vi "Invoice History.vi"(11 "reference in":T1) -> (3 "reference out":T1)   [LabVIEW 2017]
uses:
  <vilib>/addons/database/Connection.llb/Conn ObjectReference.ctl
  Control/State machine.ctl
  <vilib>/Utility/miscctls.llb/LVPointTypeDef.ctl
  8dd361f1-169d-4dbd-a915-f8e7e06827b6.vi
  <vilib>/Array/Sort 2D Array - Pop Stack.vi
  <vilib>/Array/Sort 2D Array - Push Stack.vi
  <vilib>/addons/database/Connection.llb/Conn Execute.vi
  <vilib>/addons/database/Recordset.llb/Rec Fetch Recordset Data (R).vi
  <vilib>/addons/database/Recordset.llb/Rec Destroy - Connection.vi
  <vilib>/addons/database/_DB Variant To Data/Database Variant To Data.xnode
  <vilib>/addons/database/NI_Database_API.lvlib
panel:
  in  "Search":string(combo)
  in  "Invoice CODE":string(combo)
  out "Invoice Date":timestamp format="%<%d/%m/%Y>T"
  out "Table":string[][](table)
  # "INVOICE HISTORY"
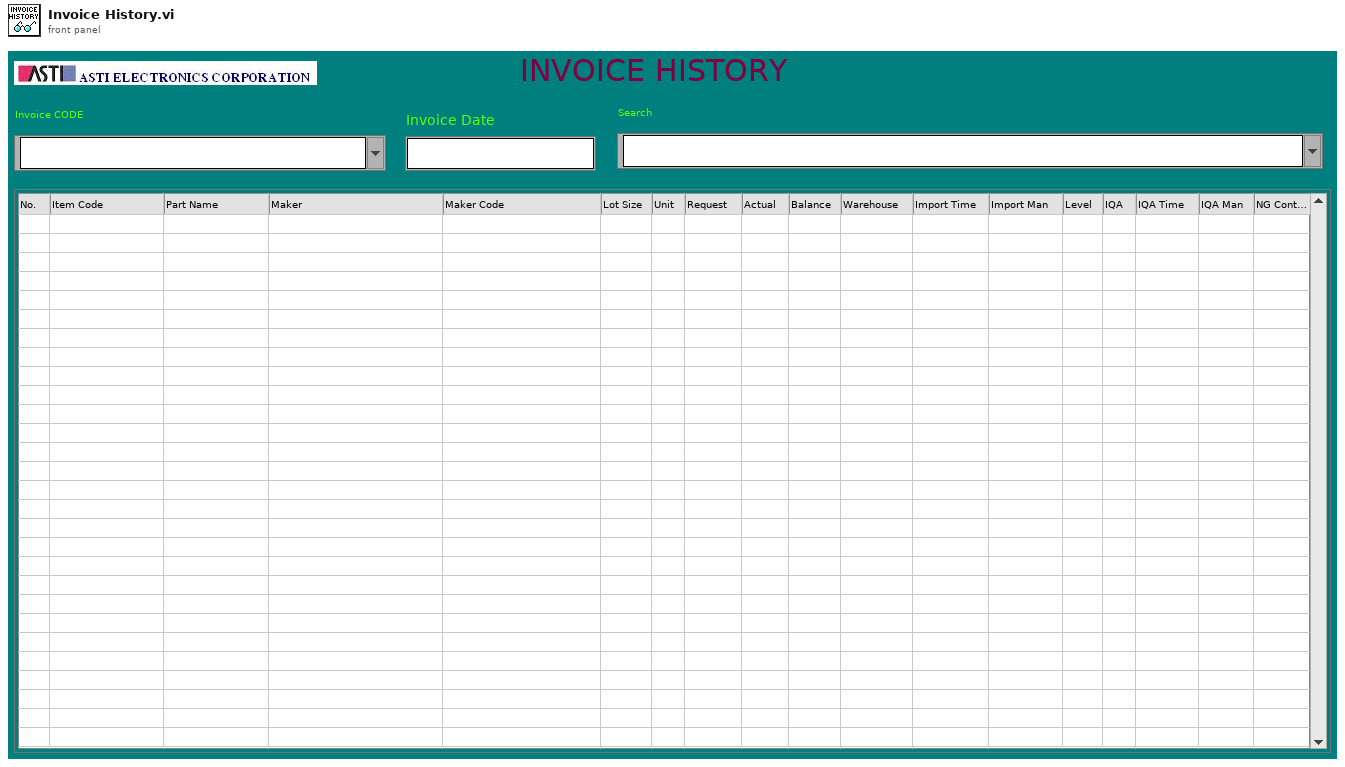
[diagram p1: front panel]
types:
  T1 = typedef "NI_Database_API.lvlib/Conn ObjectReference.ctl" = refnum<k1>
  T2 = typedef "LVPointTypeDef.ctl" = cluster{"Horizontal":i16, "Vertical":i16}
  T3 = typedef "State machine.ctl" = enum16{"Licence check", "Initial", "Log in", "Creat Config file", "Network setting", "Creat database 1", "Creat database 2", "Creat database 3", "Transfer", "Begin", "Exit"}
  T4 = typedef "NI_Database_API.lvlib/Rec ObjectReference.ctl" = refnum<k1>
  T5 = cluster{"[0]":string, "[1]":string, "[2]":string, "[3]":string, "[4]":string, "[5]":string, "[6]":string, "[7]":string, "[8]":string, "[9]":string, "[10]":string, "[11]":string, "[12]":string, "[13]":string, "[14]":string, "[15]":string}
  T6 = cluster{"[0]":string, "[1]":string, "[2]":string, "[3]":string, "[4]":string, "[5]":string, "[6]":string, "[7]":string, "[8]":string, "[9]":string, "[10]":string, "[11]":string, "[12]":string, "[13]":string, "[14]":string, "[15]":string}[]
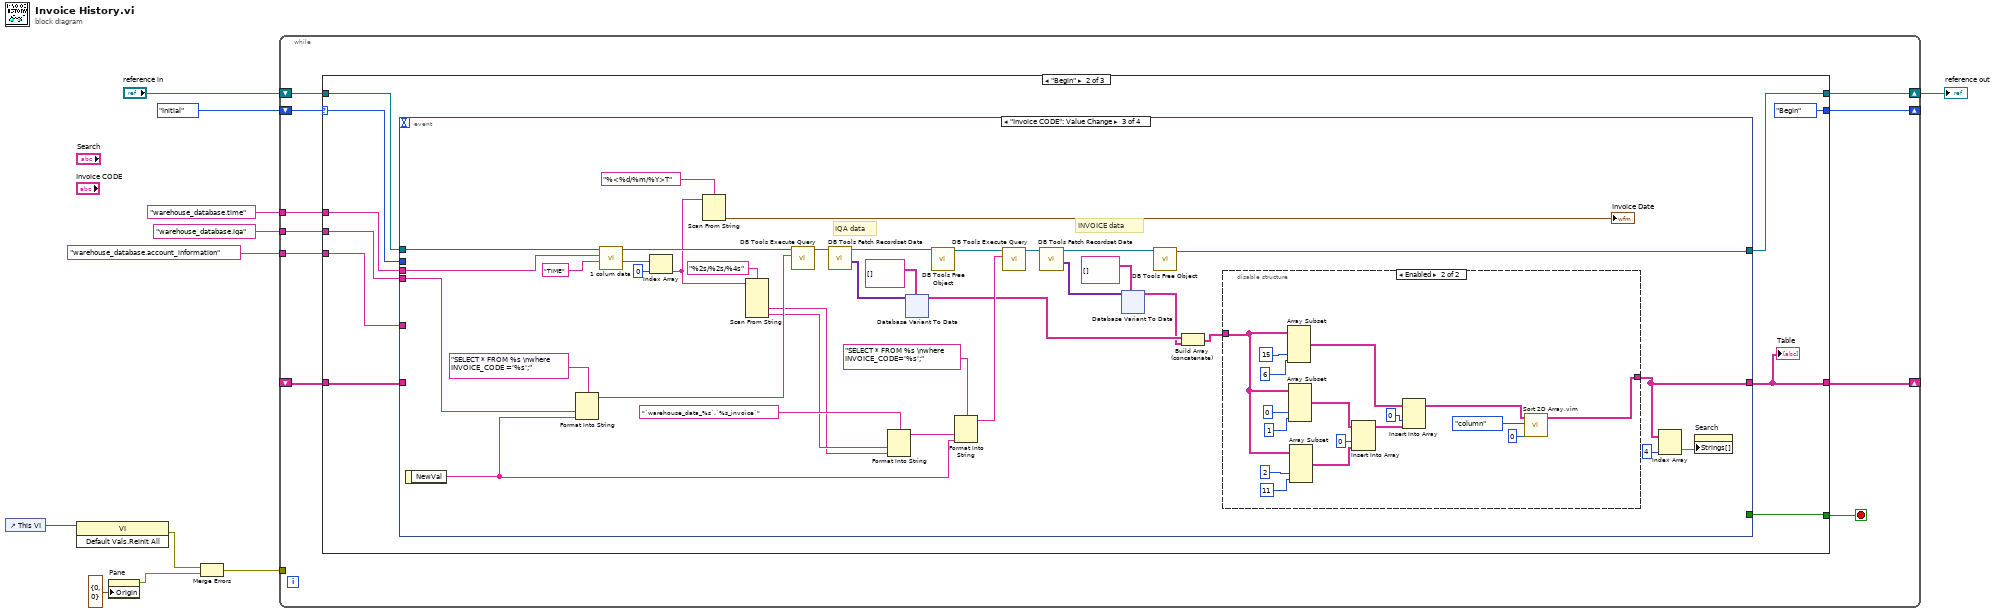
[diagram p0: block diagram]
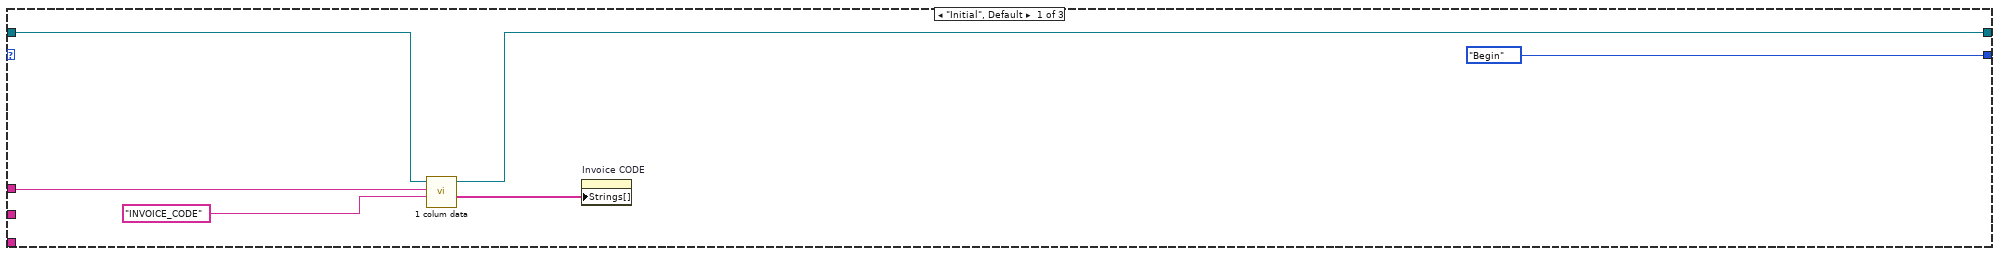
[diagram p2: hidden frame]
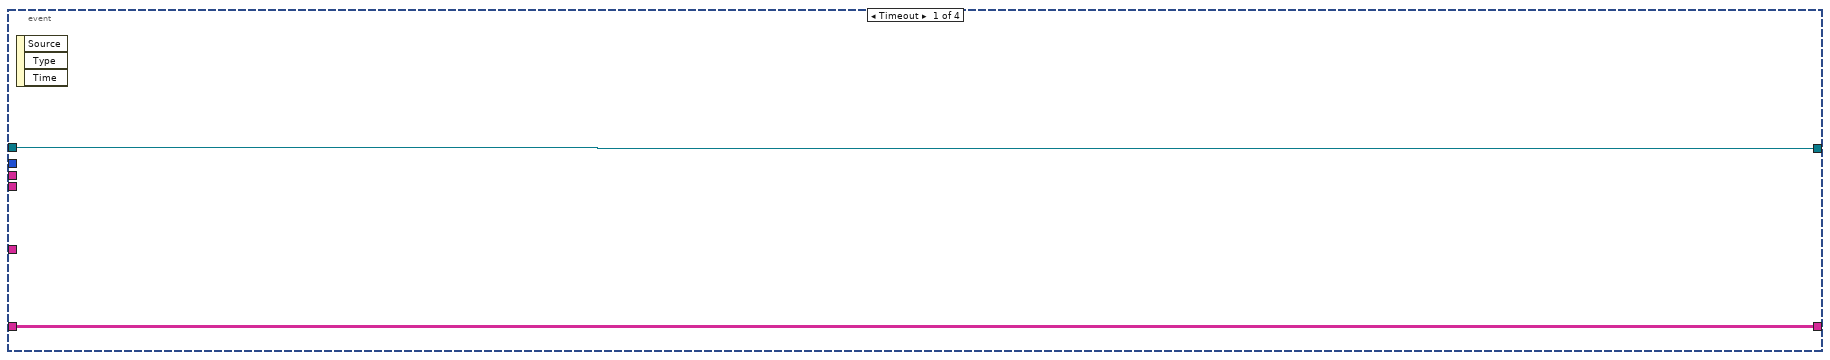
[diagram p3: hidden frame]
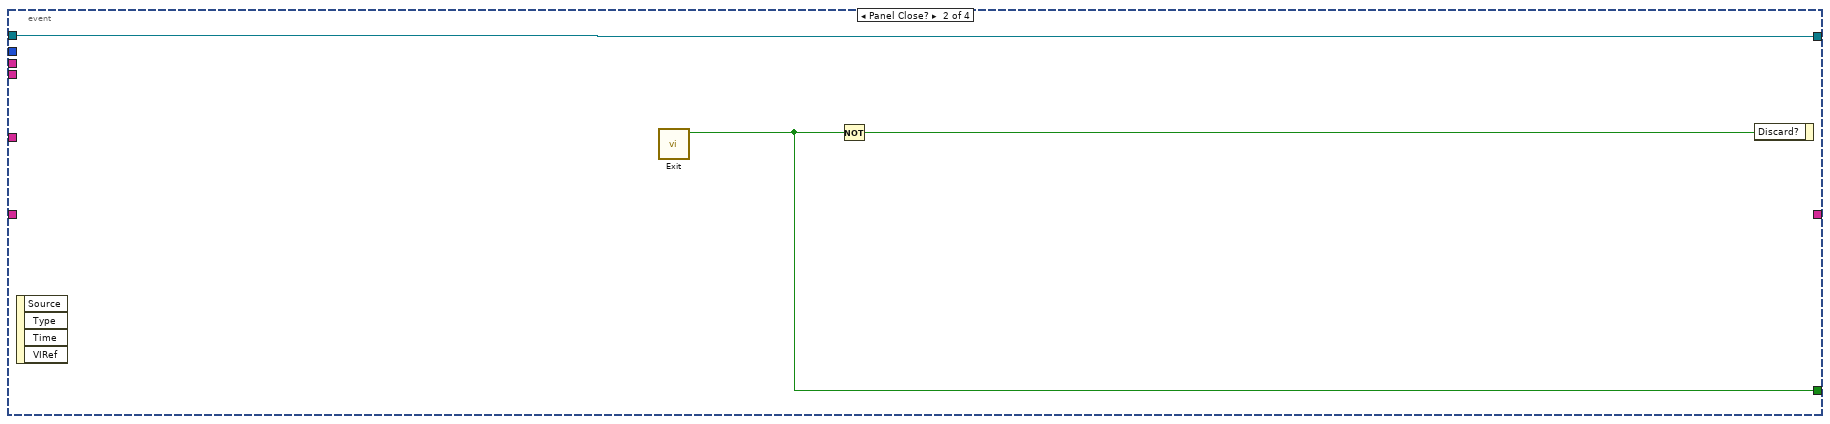
[diagram p4: hidden frame]
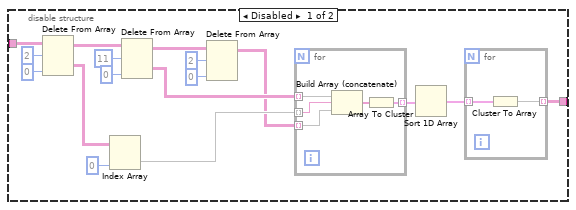
[diagram p5: hidden frame]
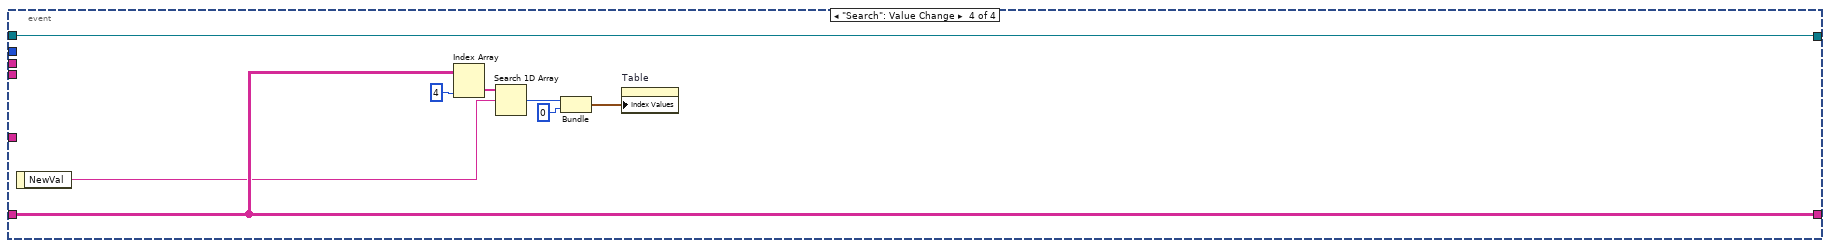
[diagram p6: hidden frame]
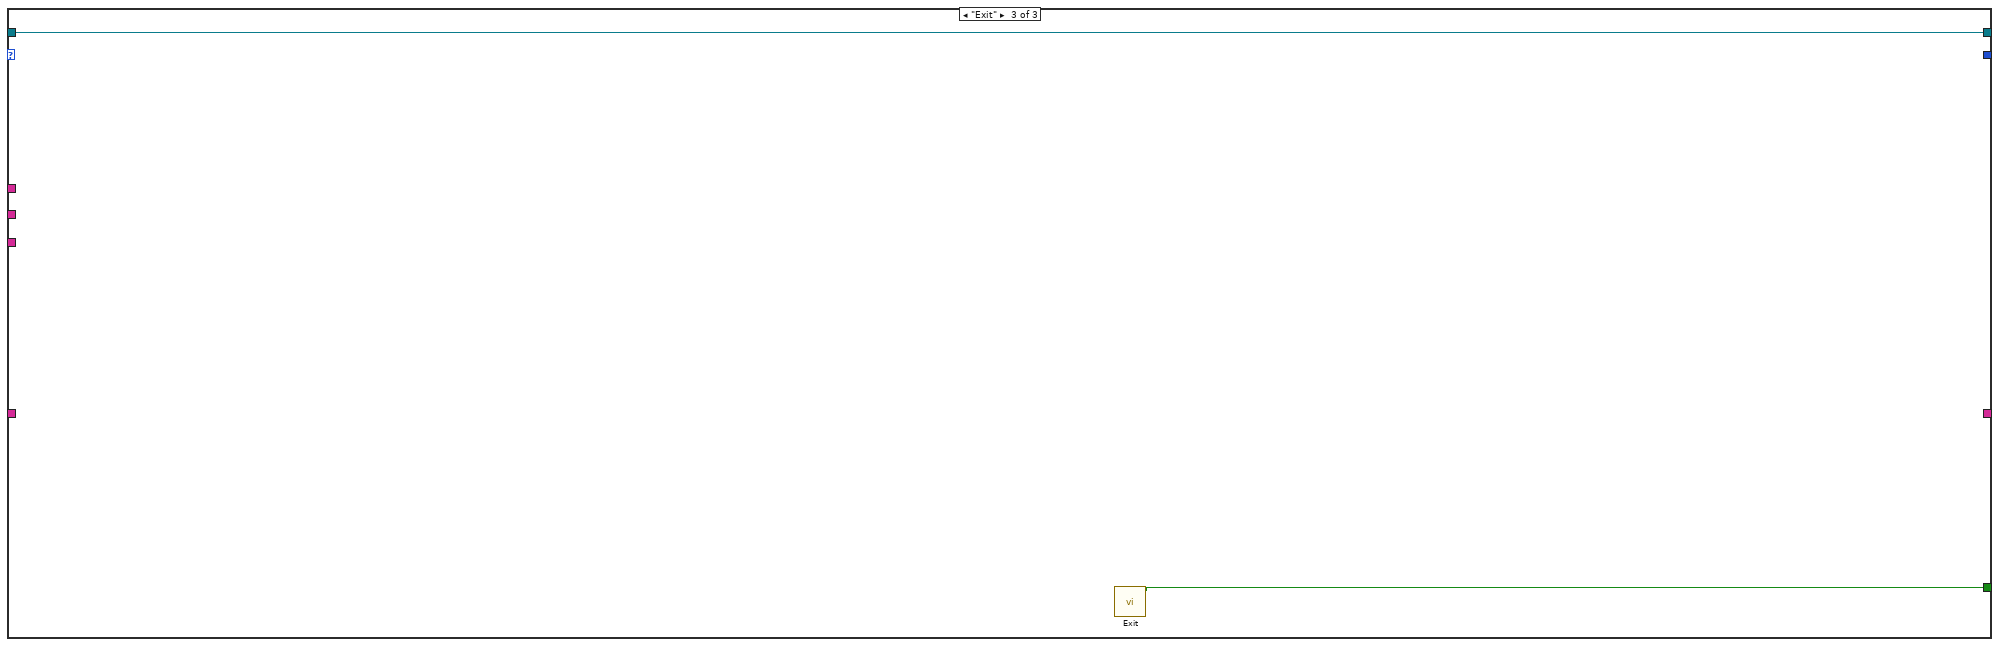
[diagram p7: hidden frame]
diagram:
  n1 = control-ref of="This VI"() -> (w10:refnum<vi>)
  n2 = invoke class="VI" method="Default Vals.Reinit All"(reference=w10) -> (error out=w8:errorcluster)  [unwired: 2 in, 2 out]
  n3 = property on="Pane" class="Pane"("Origin"=T2 {"Horizontal"=0, "Vertical"=0}) -> (error out=w7:errorcluster)  [unwired: 2 in, 1 out]
  n4 = Merge Errors(w8, w7) -> (w6:errorcluster)
  n5 = while {
    shift-right: [w19] -> _
    shift-left: State_machine."Initial" ("Enum") -> [w20]
    shift-right: [w18] -> w1
    shift-left: "reference in" -> [w17]
    tunnel: w6 -> [_]
    tunnel: "warehouse_database.time" ("table") -> [w16]
    tunnel: "warehouse_database.iqa" ("table") -> [w15]
    tunnel: "warehouse_database.account_information" -> [w14]
    shift-right: [w13] -> _
    shift-left: _ -> [w12]
    stop <- w21 stop-if-true
    n6 = case shown="\"Begin\"" w20 {
      selector: w20 -> [_ w34 _]
      tunnel: [_ w37 w216] -> w21
      tunnel: [State_machine."Begin" ("Enum") State_machine."Begin" ("Enum") _] -> w19
      tunnel: [w25 w35 w217] -> w18
      tunnel: w17 -> [w26 w36 w217]
      tunnel: w16 -> [w22 w32 _]
      tunnel: w15 -> [_ w31 _]
      tunnel: w14 -> [_ w30 _]
      tunnel: [_ w29 _] -> w13
      tunnel: w12 -> [_ w28 _]
      frame "Initial", Default {
        n7 = call "1 colum data.vi"("column"="INVOICE_CODE" ("String"), "table"=w22, "Refnum in"=w26) -> ("data"=w23:string[], "Refnum out"=w25:T1)  [unwired: 6 in, 1 out]
        n8 = property on="Invoice CODE" class="CmbBox"("Strings[]"=w23) -> ()  [unwired: 2 in, 2 out]
      }
      frame "Begin" {
        n9 = event shown="[2] \"Invoice CODE\": Value Change" {
          selector: _ -> [_ _ _ _]
          dyn-events: _ -> [_ _ _ _]
          timeout: _ -> [_ _ _ _]
          tunnel: [_ w42 _ _] -> w37
          tunnel: w36 -> [w39 w40 w78 w208]
          tunnel: [w39 w40 w62 w208] -> w35
          tunnel: w34 -> [_ _ _ _]
          tunnel: w32 -> [_ _ w77 _]
          tunnel: w31 -> [_ _ w67 _]
          tunnel: w30 -> [_ _ _ _]
          tunnel: [w38 _ w43 w210] -> w29
          tunnel: w28 -> [w38 _ _ w210]
          event Timeout {
            n10 = event-data() -> ()  [unwired: 1 in, 3 out]
          }
          event Panel Close? {
            n11 = event-data() -> ()  [unwired: 1 in, 4 out]
            n12 = call "Exit.vi"() -> ("T button?"=w42:bool)  [unwired: 11 in]
            n13 = Not(x=w42) -> (.not. x?=w41:bool)
            n14 = event-data("Discard?"=w41) -> ()  [unwired: 1 in, 1 out]
          }
          event "Invoice CODE": Value Change {
            # "INVOICE data"
            # "IQA data"
            n15 = event-data() -> ("NewVal"=w59:string)  [unwired: 1 in]
            n16 = Format Into String(format string="SELECT * FROM %s \nwhere INVOICE_CODE ='%s';", w67, w59) -> (resulting string=w66:string)  [unwired: 2 in, 1 out]
            n17 = call "1 colum data.vi"("column"="TIME", "table"=w77, "Refnum in"=w78) -> ("data"=w75:string[], "Refnum out"=w72:T1)  [unwired: 6 in, 1 out]
            n18 = Index Array(array=w75, index=0) -> (element=w53:string)
            n19 = Scan From String(format string="%<%d/%m/%Y>T", input string=w53) -> (output 1=→"Invoice Date":timestamp)  [unwired: 3 in, 3 out]
            n20 = Scan From String(format string="%2s/%2s/%4s", input string=w53) -> (output 2=w46:string, output 3=w47:string)  [unwired: 6 in, 3 out]
            n21 = call-poly <vilib>:"DB Tools Execute Query.vi"("SQL query"=w66, "connection reference"=w72) -> ("recordset reference"=w71:T4)  [unwired: 6 in, 1 out]
            n22 = call-poly <vilib>:"DB Tools Fetch Recordset Data.vi"("recordset reference"=w71) -> ("recordset data"=w69:variant[][], "recordset reference out"=w70:T4)  [unwired: 4 in, 1 out]
            n23 = Format Into String(format string="`warehouse_data_%s`.`%s_invoice`" ("string"), w47, w46) -> (resulting string=w45:string)  [unwired: 2 in, 1 out]
            n24 = xnode "Database Variant To Data"("database variant"=w69, "type"=string[][] []) -> ("data"=w55:string[][])  [unwired: 1 in, 1 out]
            n25 = call-poly <vilib>:"DB Tools Free Object.vi"("recordset reference"=w70) -> ("connection reference"=w63:T1)  [unwired: 9 in, 1 out]
            n26 = Format Into String(format string="SELECT * FROM %s \nwhere INVOICE_CODE='%s';", w45, w59) -> (resulting string=w58:string)  [unwired: 2 in, 1 out]
            n27 = call-poly <vilib>:"DB Tools Execute Query.vi"("SQL query"=w58, "connection reference"=w63) -> ("recordset reference"=w64:T4)  [unwired: 6 in, 1 out]
            n28 = call-poly <vilib>:"DB Tools Fetch Recordset Data.vi"("recordset reference"=w64) -> ("recordset data"=w56:variant[][], "recordset reference out"=w65:T4)  [unwired: 4 in, 1 out]
            n29 = xnode "Database Variant To Data"("database variant"=w56, "type"=string[][] []) -> ("data"=w54:string[][])  [unwired: 1 in, 1 out]
            n30 = call-poly <vilib>:"DB Tools Free Object.vi"("recordset reference"=w65) -> ("connection reference"=w62:T1)  [unwired: 9 in, 1 out]
            n31 = Build Array (concatenate)(w55, w54) -> (w44:string[][])
            n32 = disable-structure shown="Enabled" {
              disable-tunnel: w44 -> [w79 w107]
              disable-tunnel: [w80 w119] -> w43
              frame Disabled {
                n33 = Delete From Array(array=w79, length=2, index (col)=0 ("disabled index (col)")) -> (deleted portion=w87:string[][], array with subset deleted=w93:string[][])  [unwired: 1 in]
                n34 = Index Array(array=w87, index (col)=0 ("disabled index (col)")) -> (element=w84:string[])  [unwired: 1 in]
                n35 = Delete From Array(array=w93, length=11, index (col)=0 ("disabled index (col)")) -> (deleted portion=w85:string[][], array with subset deleted=w88:string[][])  [unwired: 1 in]
                n36 = Delete From Array(array=w88, length=2, index (col)=0 ("disabled index (col)")) -> (array with subset deleted=w83:string[][])  [unwired: 1 in, 1 out]
                n37 = for {
                  tunnel: w85 -> [w102] mode=indexing
                  tunnel: w84 -> [w101] mode=indexing
                  tunnel: w83 -> [w100] mode=indexing
                  tunnel: [w98] -> w82 mode=indexing
                  n38 = Build Array (concatenate)(w102, w101, w100) -> (w99:string[])
                  n39 = Array To Cluster(array=w99) -> (cluster=w98:T5)
                }
                n40 = Sort 1D Array(array=w82) -> (sorted array=w81:T6)
                n41 = for {
                  tunnel: w81 -> [w97] mode=indexing
                  tunnel: [w96] -> w80 mode=indexing
                  n42 = Cluster To Array(cluster=w97) -> (array=w96:string[])
                }
              }
              frame Enabled {
                n43 = Array Subset(array=w107, index (col)=15 ("index"), length (col)=6 ("length")) -> (w105:string[][])  [unwired: 2 in]
                n44 = Array Subset(array=w107, index (col)=0 ("index"), length (col)=1 ("length")) -> (w112:string[][])  [unwired: 2 in]
                n45 = Array Subset(array=w107, index (col)=2 ("index"), length (col)=11 ("length")) -> (w111:string[][])  [unwired: 2 in]
                n46 = Insert Into Array(array=w112, index (col)=0 ("disabled index (col)"), new element=w111) -> (w104:string[][])  [unwired: 1 in]
                n47 = Insert Into Array(array=w105, index (col)=0 ("disabled index (col)"), new element=w104) -> (w103:string[][])  [unwired: 1 in]
                n48 = call "Sort 2D Array.vim"("index"=0, "dimension to index (column)"=enum16{"column", "row"}."column", "2D array"=w103) -> ("sorted 2D array"=w119:string[][])  [unwired: 7 in, 1 out]
              }
            }
            n49 = Index Array(array=w43, index (col)=4 ("disabled index (col)")) -> (element=w49:string[])  [unwired: 1 in]
            n50 = property on="Search" class="CmbBox"("Strings[]"=w49) -> ()  [unwired: 2 in, 2 out]
          }
          event "Search": Value Change {
            n51 = event-data() -> ("NewVal"=w209:string)  [unwired: 1 in]
            n52 = Index Array(array=w210, index (col)=4 ("disabled index (col)")) -> (element=w212:string[])  [unwired: 1 in]
            n53 = Search 1D Array(1D array=w212, element=w209) -> (index of element=w215:i32)  [unwired: 1 in]
            n54 = Bundle("index of element"=w215, 0) -> (w214:cluster{"index of element":i32, i32})  [unwired: 1 in]
            n55 = property on="Table" class="Tbl (strict)"("Index Values"=w214) -> ()  [unwired: 2 in, 2 out]
          }
        }
        "Table" <- w29
      }
      frame "Exit" {
        n56 = call "Exit.vi"() -> ("T button?"=w216:bool)  [unwired: 11 in]
      }
    }
  }
  "reference out" <- w1
